vi "Hardware Test.vi"() -> ()   [LabVIEW 2019]
uses:
  <vilib>/FPGAPlugInAG/myRIO-1900/niLvFpga_Open_myRIO-1900.vi
  <vilib>/rvi/interface/common/dynamic/niFpgaDynamicAddResources.vi
  <vilib>/Utility/error.llb/Error Cluster From Error Code.vi
  <vilib>/rvi/errors/niLvFpgaAdjustHostInterfaceError.vi
  <vilib>/FPGAPlugInAG/Dynamic/niLvFpga_Close_Dynamic.vi
  <vilib>/rvi/interface/nirviOpenFPGA/nirviOpenFPGA.xnode
  FPGA Bitfiles/MRmecanum_FPGATarget_FPGAMainModified_TerasRobot_LKSN2021.lvbitx
  <vilib>/rvi/interface/nirviReadWriteControl/nirviReadWriteControl.xnode
  <vilib>/rvi/interface/nirviCloseFPGA/nirviCloseFPGA.xnode
  <vilib>/rvi/interface/Simulation/niFpgaSimulationCallBeginRW.vi
  NiFpgaLv.dll
panel:
  out "LIMIT SWITCH 1":bool
  out "START BUTTON":bool
  in  "M5":i16(slide) scale=-4000.0..4000.0
  out "ENC M5":i32
  in  "SERVO 4":u16(slide)=3750 scale=1000.0..6500.0
  in  "SERVO 3":u16(slide)=3750 scale=1000.0..6500.0
  in  "SERVO 2":u16(slide)=3750 scale=1000.0..6500.0
  in  "SERVO 1":u16(slide)=3750 scale=1000.0..6500.0
  out "IR 8":u16(slide) scale=0.0..2000.0
  out "IR 7":u16(slide) scale=0.0..2000.0
  out "IR 6":u16(slide) scale=0.0..2000.0
  out "IR 5":u16(slide) scale=0.0..2000.0
  in  "M4":i16(slide) scale=-4000.0..4000.0
  in  "M3":i16(slide) scale=-4000.0..4000.0
  in  "M2":i16(slide) scale=-4000.0..4000.0
  in  "M1":i16(slide) scale=-4000.0..4000.0
  out "ENC M4":i32
  out "ENC M3":i32
  out "ENC M2":i32
  out "ENC M1":i32
  out "LINE 2":bool
  out "LINE 1":bool
  out "IR 4":u16(slide) scale=0.0..2000.0
  out "IR 3":u16(slide) scale=0.0..2000.0
  out "IR 2":u16(slide) scale=0.0..2000.0
  out "IR 1":u16(slide) scale=0.0..2000.0
  in  "stop":bool
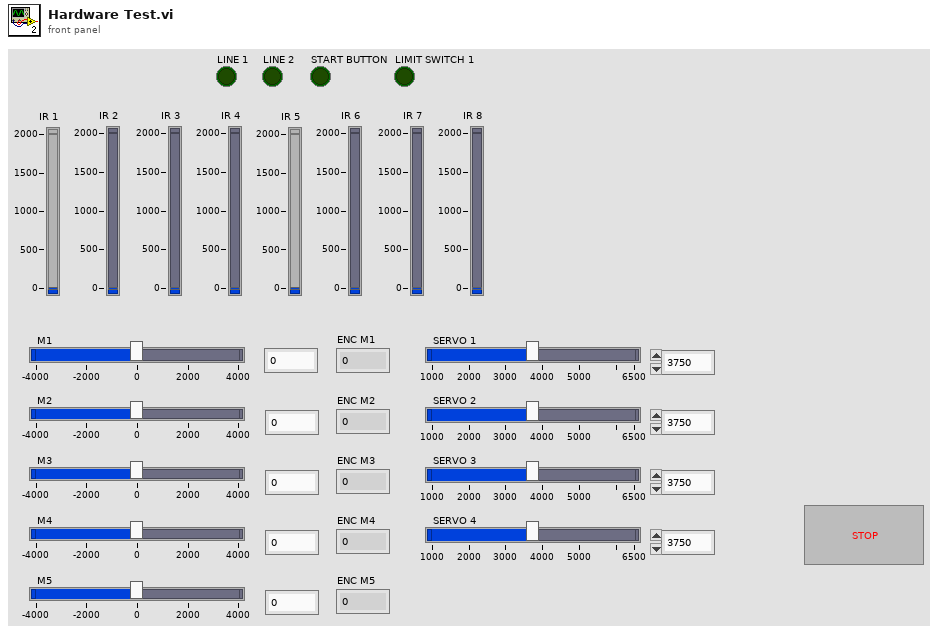
[diagram p1: front panel]
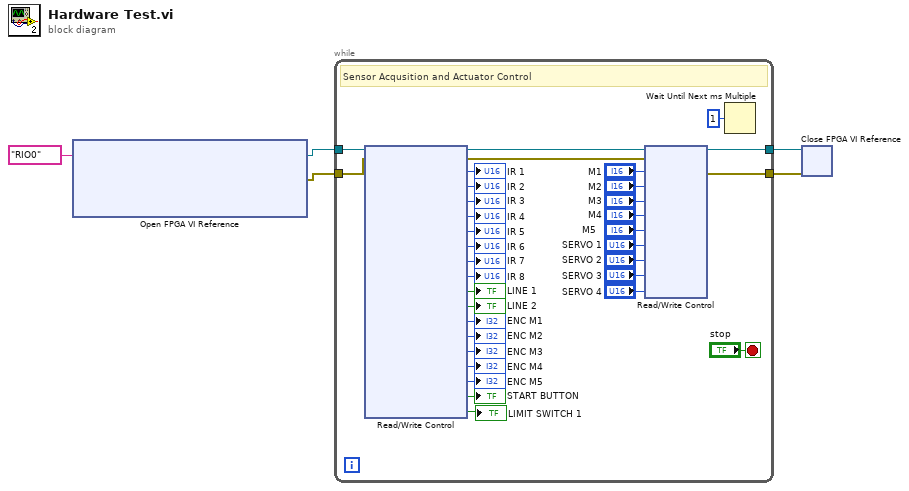
[diagram p0: block diagram]
diagram:
  n1 = xnode "Open FPGA VI Reference"("resource name"=tag "RIO0") -> ("FPGA VI Reference Out"=w4:refnum<k20>, "error out"=w5:errorcluster)  [unwired: 1 in]
  n2 = while {
    tunnel: w5 -> [w37]
    tunnel: w4 -> [w38]
    tunnel: [w25] -> w3
    tunnel: [w19] -> w2
    stop <- "stop" stop-if-true
    # "Sensor Acqusition and Actuator Control"
    n3 = xnode "Read/Write Control"("FPGA VI Reference In"=w38, "error in"=w37) -> ("FPGA VI Reference Out"=w36:refnum<k20>, "error out"=w20:errorcluster, "IR 1"=→"IR 1":u16, "IR 2"=→"IR 2":u16, "IR 3"=→"IR 3":u16, "IR 4"=→"IR 4":u16, "IR 5"=→"IR 5":u16, "IR 6"=→"IR 6":u16, "IR 7"=→"IR 7":u16, "IR 8"=→"IR 8":u16, "LINE 1"=→"LINE 1":bool, "LINE 2"=→"LINE 2":bool, "ENC M1"=→"ENC M1":i32, "ENC M2"=→"ENC M2":i32, "ENC M3"=→"ENC M3":i32, "ENC M4"=→"ENC M4":i32, "ENC M5"=→"ENC M5":i32, "START BUTTON"=→"START BUTTON":bool, "LIMIT SWITCH 1"=→"LIMIT SWITCH 1":bool)
    n4 = xnode "Read/Write Control"("FPGA VI Reference In"=w36, "error in"=w20, "M1"="M1", "M2"="M2", "M3"="M3", "M4"="M4", "M5"="M5", "SERVO 1"="SERVO 1", "SERVO 2"="SERVO 2", "SERVO 3"="SERVO 3", "SERVO 4"="SERVO 4") -> ("FPGA VI Reference Out"=w25:refnum<k20>, "error out"=w19:errorcluster)
    n5 = Wait Until Next ms Multiple(millisecond multiple=u32 1) -> ()  [unwired: 1 out]
  }
  n6 = xnode "Close FPGA VI Reference"("FPGA VI Reference In"=w3, "error in"=w2) -> ()  [unwired: 1 out]
